vi "Trigger Pattern Query.vi"(8 "error in":errorcluster, 11 "Instrument Handle In":i32) -> (0 "error out":errorcluster, 1 "Pattern Truth":i32, 2 "Pattern Mask":i32, 3 "Instrument Handle Out":i32, 4 "Type":i32 caption="Pattern Type")   [LabVIEW 8.6, in "ZTScopeM.lvlib"]
doc: "Query the pattern triggering configuration"
uses:
  ZTScopeM.lvlib
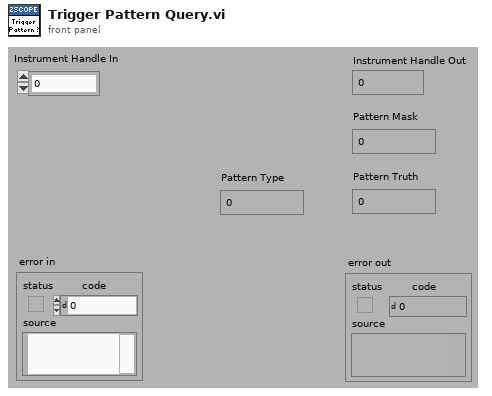
[diagram p1: front panel]
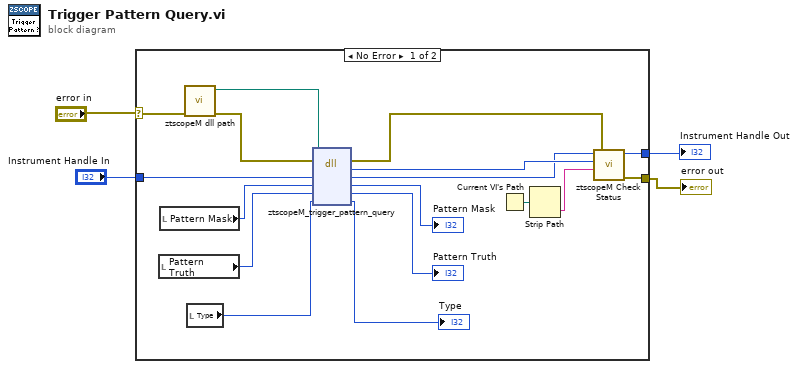
[diagram p0: block diagram]
diagram:
  n1 = case shown="No Error" "error in" {
    selector: "error in" -> [w8 w23]
    tunnel: [w12 w23] -> w1
    tunnel: "Instrument Handle In" -> [w21 w22]
    tunnel: [w11 w22] -> w3
    frame #0 {
      n2 = local read "Pattern Truth"() -> (w18:i32)
      n3 = local read "Pattern Mask"() -> (w20:i32)
      n4 = call "ztscopeM dll path.vi"("error in (no error)"=w8) -> ("error out"=w6:errorcluster, "<instrument>.dll path"=w7:path)  [unwired: 9 in]
      n5 = local read "Type"() -> (w9:i32)
      n6 = dll-call lib="C:/Program Files (x86)/National Instruments/LabVIEW 2013/instr.lib/ztscopem/ztscopeM.dll" fn="ztscopeM_trigger_pattern_query"(path in=w7, error in=w6, "instrumentHandle"=w21, "patternMask"=w20, "patternTruth"=w18, "type"=w9) -> (error out=w5:errorcluster, w14:i32, "instrumentHandle"=w13:i32, "patternMask"=→"Pattern Mask":i32, "patternTruth"=→"Pattern Truth":i32, "type"=→"Type":i32)  [unwired: 1 in, 1 out]
      n7 = Current VI's Path() -> (path=w16:path)
      n8 = Strip Path(path=w16) -> (name=w15:string)  [unwired: 1 out]
      n9 = call "ztscopeM Check Status.vi"("error in"=w5, "name of VI"=w15, "status (return code)"=w14, "instrument handle in"=w13) -> ("error out"=w12:errorcluster, "instrument handle out"=w11:i32)  [unwired: 2 in]
    }
    frame #1 {
    }
  }
  "Instrument Handle Out" <- w3
  "error out" <- w1
